vi "AFM.DLog.Create.vi"(8 "error in (no error)":errorcluster, 11 "Instrument.AFM_DLog in":refnum<class "Instrument.AFM_DLog.lvclass">) -> (0 "error out":errorcluster, 2 "Public Events":T1, 3 "Instrument.AFM_DLog out":refnum<class "Instrument.AFM_DLog.lvclass">)   [LabVIEW 2019, in "Instrument.AFM_DLog.lvclass"]
uses:
  Instrument.AFM_DLog.lvclass
  <userlib>/LevyLab/Instrument Framework/Instrument/Instrument.lvclass
  <vilib>/JKI/JKI SMO/SMO/SMO.lvclass
  <vilib>/JKI/JKI SMO/SMO/Typedefs/SMOState --Enum.ctl
  C:/Program Files (x86)/National Instruments/LabVIEW 2019/user.lib/LevyLab/Instrument Framework/Instrument Types/SCPI/Instrument.SCPI.lvclass
  C:/Program Files (x86)/National Instruments/LabVIEW 2019/user.lib/LevyLab/Instrument Framework/Instrument/Instrument.lvclass
  C:/Program Files (x86)/National Instruments/LabVIEW 2019/vi.lib/JKI/JKI SMO/SMO/SMO.lvclass
  <userlib>/LevyLab/RemoteControl/RemoteControl/Typedefs/Message--Cluster.ctl
  <userlib>/LevyLab/RemoteControl/RemoteControl/RemoteControl.lvclass
  Typedefs/PublicEvents--AFM_DLog.MessageFromProcess.ctl
  Typedefs/PublicEvents--Cluster.ctl
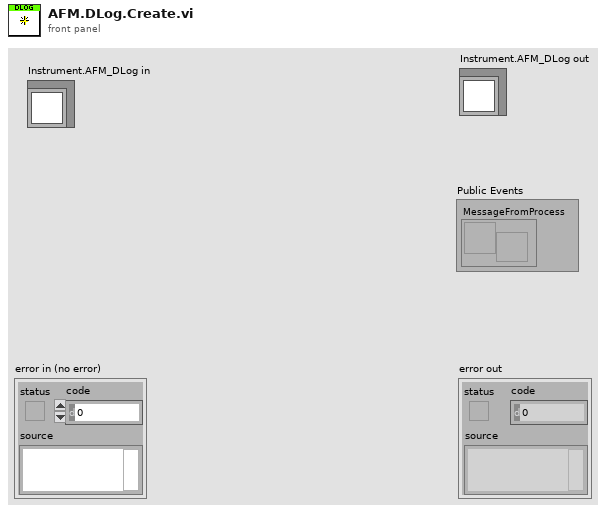
[diagram p1: front panel]
types:
  T1 = typedef "Instrument.AFM_DLog.lvclass/PublicEvents--Cluster.ctl" = cluster{"MessageFromProcess":refnum<user-event>}
  T2 = typedef "smo.lvlib/SMO.lvclass/SMOState --Enum.ctl" = enum16{"unknown", "Created", "Started", "Stopped"}
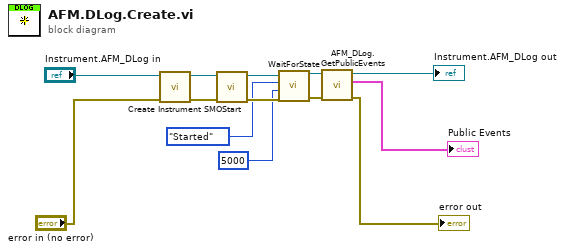
[diagram p0: block diagram]
diagram:
  n1 = call <userlib>:"Create Instrument SMO.vi"("error in (no error)"="error in (no error)", "Instrument in"="Instrument.AFM_DLog in") -> ("error out"=w11:errorcluster, "Instrument out"=w13:refnum<class "Instrument.AFM_DLog.lvclass">)  [unwired: 8 in]
  n2 = call <vilib>:"Start.vi"("error in (no error)"=w11, "SMO"=w13) -> ("error out"=w10:errorcluster, "SMO out"=w12:refnum<class "Instrument.AFM_DLog.lvclass">)  [unwired: 8 in]
  n3 = call <vilib>:"WaitForState.vi"("error in (no error)"=w10, "timeout in ms (-1)"=5000, "State (unknown: any state)"=SMOState_--Enum."Started" ("SMO State"), "SMO in"=w12) -> ("error out"=w4:errorcluster, "SMO out"=w5:refnum<class "Instrument.AFM_DLog.lvclass">)  [unwired: 5 in, 1 out]
  n4 = call "AFM_DLog.GetPublicEvents.vi"("error in (no error)"=w4, "Instrument.AFM_DLog in"=w5) -> ("error out"=→"error out":errorcluster, "Public Events"=→"Public Events":T1, "Instrument.AFM_DLog out"=→"Instrument.AFM_DLog out":refnum<class "Instrument.AFM_DLog.lvclass">)  [unwired: 7 in]
